vi "Write Voltage.vi"(8 "error in (no error)":errorcluster, 10 "Voltage":sgl, 11 "HVPS in":refnum<class "HVPS.lvclass">) -> (0 "error out":errorcluster, 3 "HVPS out":refnum<class "HVPS.lvclass">)   [LabVIEW 2013, in "HVPS.lvclass"]
uses:
  HVPS.lvclass
  HVPS.lvclass/HVPS.ctl
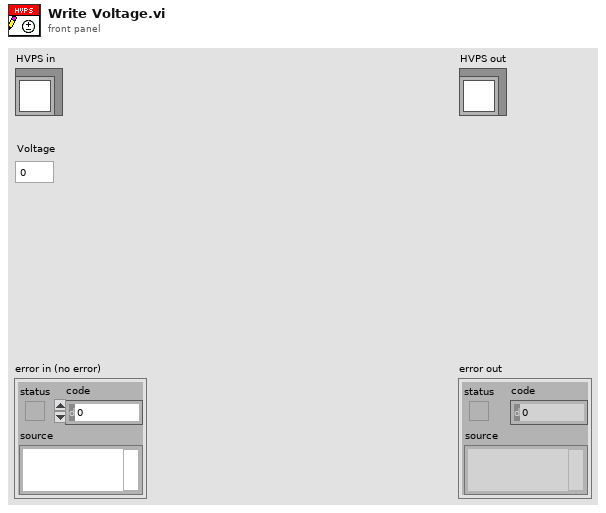
[diagram p1: front panel]
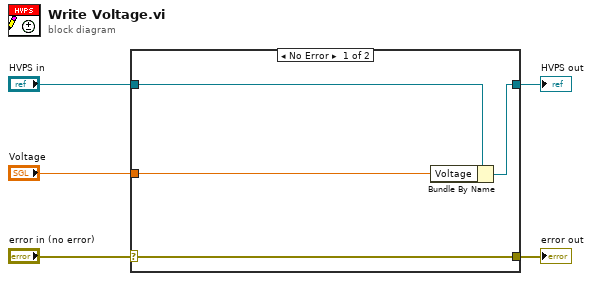
[diagram p0: block diagram]
diagram:
  n1 = case shown="No Error" "error in (no error)" {
    selector: "error in (no error)" -> [w9 w10]
    tunnel: [w9 w10] -> w4
    tunnel: [w7 w11] -> w2
    tunnel: "HVPS in" -> [w8 w11]
    tunnel: "Voltage" -> [w6 _]
    frame No Error {
      n2 = Bundle By Name(cluster=w8, "Voltage"=w6) -> (w7:refnum<class "HVPS.lvclass">)
    }
    frame Error {
    }
  }
  "error out" <- w4
  "HVPS out" <- w2
